vi "BasicMovement.vi"() -> ()   [LabVIEW 2015, in "IoTprojectg61305.lvrbt"]
uses:
  IoTprojectg61305.lvrbt
  <vilib>/NXT/Block Support/NXT_InputPort.ctl
  <vilib>/NXT/Block Support/NXT_OutputPort.ctl
  <vilib>/NXT/Dual Mode Library/Sensors/Touch_Pressed.vi
  <vilib>/NXT/Dual Mode Library/Sensors/EV3_Infrared_Proxy.vi
  <vilib>/NXT/NXTIO Xnodes/NXTIONodeSubVIs/NXTStopMotors.vi
  <vilib>/NXT/NXTIO Xnodes/NXTIONodeSubVIs/NXTMoveMotors.vi
  <vilib>/NXT/Dual Mode Library/Sound/Tone.vi
  <vilib>/NXT/Subs/LVHSConnector.ctl
  <vilib>/NXT/NXTIO Xnodes/AddressXNode/NXTIOAddress.xnode
  <vilib>/NXT/NXTIO Xnodes/NXTIOXNode/NXTIO.xnode
  <vilib>/NXT/LegoClasses/BrickReference/BrickReference.lvclass
panel:
  out "LEFT":bool
  out "STOP":bool
  out "OBSTACLE":bool
  out "posTab":i32
  in  "stop":bool
  out "RIGHT":bool
  out "new value":string
  out "old value":string
  out "UP":bool
  out "DOWN":bool
  # "Robot Modile Connecté : Lego Mindestrom EV3"
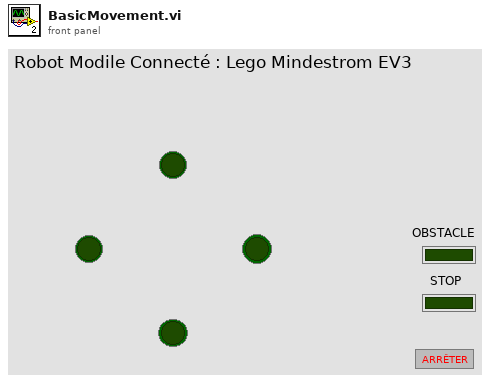
[diagram p1: front panel]
types:
  T1 = typedef "NXT_OutputPort.ctl" = u8
  T2 = typedef "NXT_InputPort.ctl" = u32
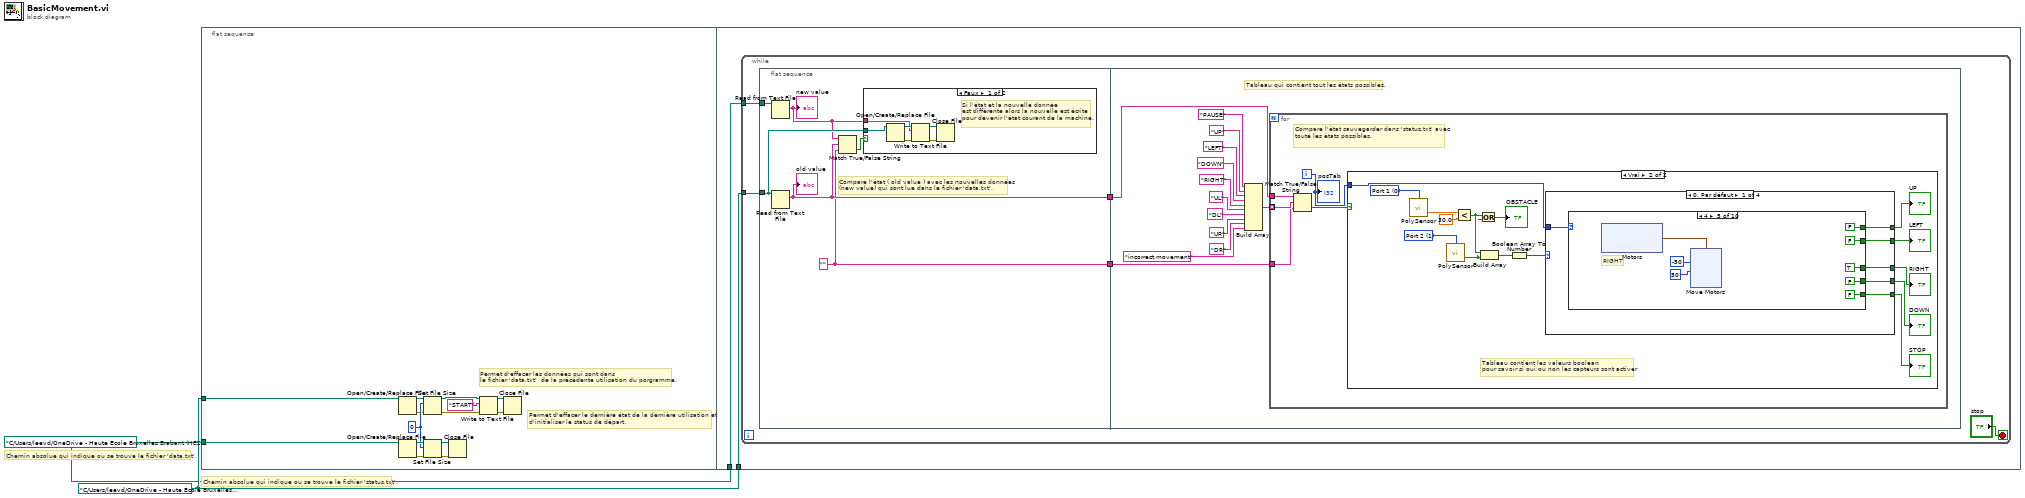
[diagram p0: block diagram]
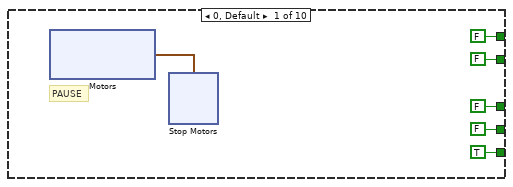
[diagram p4: hidden frame]
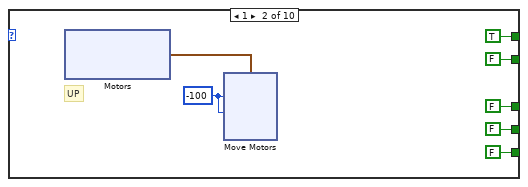
[diagram p5: hidden frame]
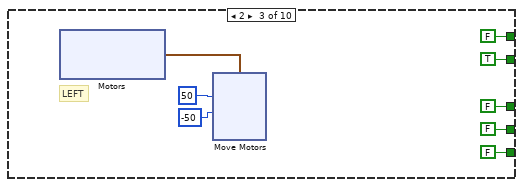
[diagram p6: hidden frame]
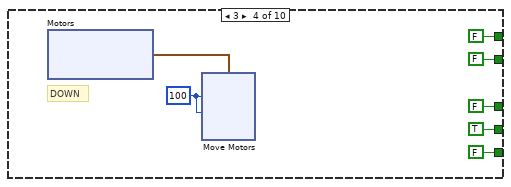
[diagram p7: hidden frame]
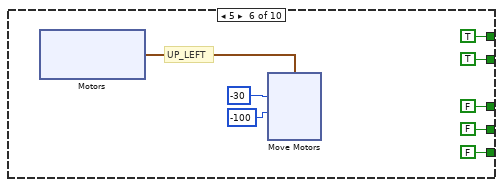
[diagram p8: hidden frame]
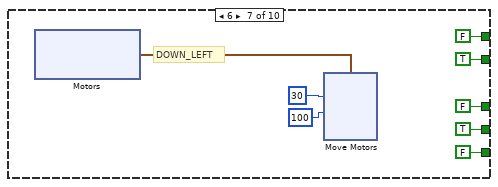
[diagram p9: hidden frame]
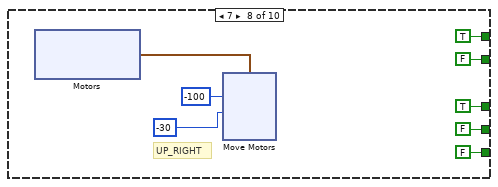
[diagram p10: hidden frame]
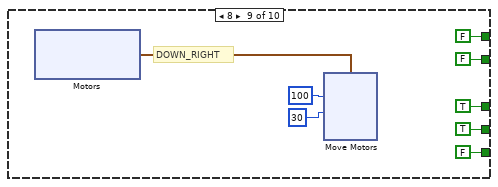
[diagram p11: hidden frame]
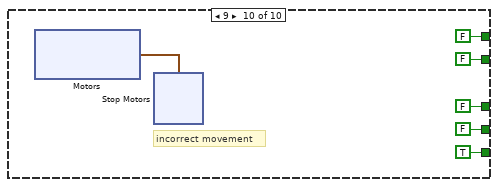
[diagram p12: hidden frame]
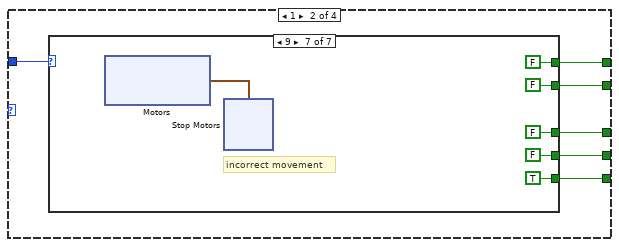
[diagram p13: hidden frame]
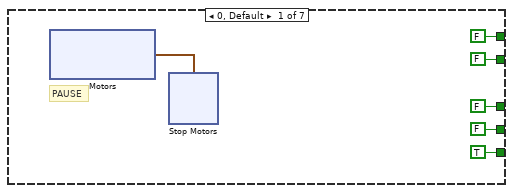
[diagram p14: hidden frame]
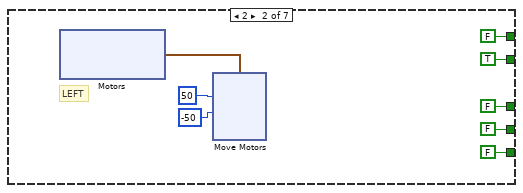
[diagram p15: hidden frame]
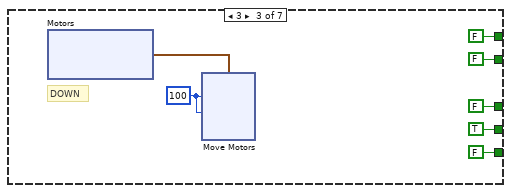
[diagram p16: hidden frame]
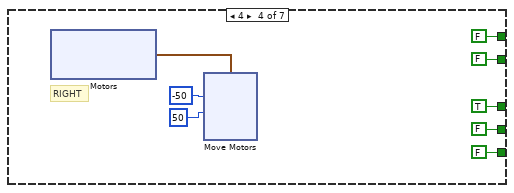
[diagram p17: hidden frame]
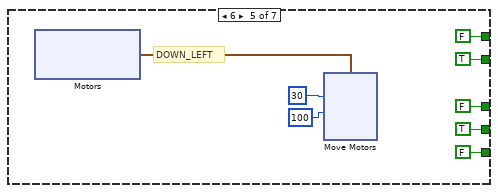
[diagram p18: hidden frame]
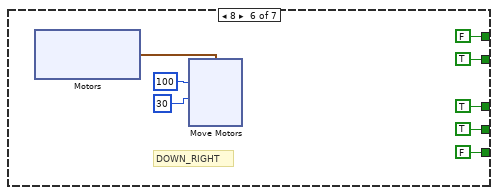
[diagram p19: hidden frame]
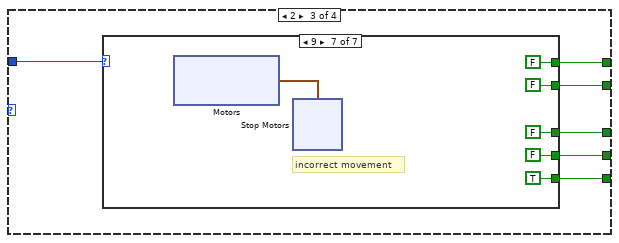
[diagram p20: hidden frame]
diagram:
  w2 = path "C:/Users/leevd/OneDrive - Haute Ecole Bruxelles Brabant (HE2B)/HE2B/Q4/IOTI4/Projet/HandTraking61305/data.txt" ("fichier (utiliser une boîte de dialogue)")
  w1 = path "C:/Users/leevd/OneDrive - Haute Ecole Bruxelles Brabant (HE2B)/HE2B/Q4/IOTI4/Projet/IoTprojectg61305/status.txt" ("fichier (utiliser une boîte de dialogue)")
  # "Chemin absolue qui indique ou se trouve le fichier 'status.txt'."
  # "Chemin absolue qui indique ou se trouve le fichier 'data.txt'."
  n1 = flat-sequence {
    tunnel: w2 -> [w9]
    tunnel: w1 -> [w8]
    tunnel: w1 -> [w17]
    tunnel: w2 -> [w18]
    frame #0 {
      w7 = i64 0 ("taille (en octets)")
      # "Permet d'effacer le dernière état de la dernière utilisation et \nd'initialiser le status de départ."
      # "Permet d'effacer les données qui sont dans \nle fichier 'data.txt'  de la précédente utilisation du porgramme."
      n2 = Open/Create/Replace File(file path (use dialog)=w9) -> (refnum out=w6:refnum<file>, error out=w3:errorcluster)  [unwired: 5 in, 1 out]
      n3 = Open/Create/Replace File(file path (use dialog)=w8) -> (refnum out=w15:refnum<file>, error out=w11:errorcluster)  [unwired: 5 in, 1 out]
      n4 = Set File Size(4:w3, 6:w7, 7:w6) -> (0:w4:errorcluster, 3:w5:refnum<file>)
      n5 = Set File Size(4:w11, 6:w7, 7:w15) -> (0:w12:errorcluster, 3:w13:refnum<file>)
      n6 = Close File(refnum=w13, error in=w12) -> ()  [unwired: 2 out]
      n7 = Write to Text File(file (use dialog)=w5, text="START", error in=w4) -> (refnum out=w14:refnum<file>, error out=w10:errorcluster)  [unwired: 1 in, 1 out]
      n8 = Close File(refnum=w14, error in=w10) -> ()  [unwired: 2 out]
    }
    frame #1 {
      n9 = while {
        tunnel: w18 -> [w22]
        tunnel: w17 -> [w21]
        stop <- "stop" stop-if-true
        n10 = flat-sequence {
          tunnel: w22 -> [w27]
          tunnel: w21 -> [w28]
          tunnel: [w25] -> w20
          tunnel: [w24] -> w19
          tunnel: w20 -> [w48]
          tunnel: w19 -> [w37]
          frame #0 {
            w24 = ""
            # "Compare l'état ( old value ) avec les nouvelles données\n(new value) qui sont lue dans le fichier 'data.txt'."
            n11 = Read from Text File(file (use dialog)=w28) -> (text=w26:string)  [unwired: 3 in, 3 out]
            "new value" <- w26
            n12 = Read from Text File(file (use dialog)=w27) -> (text=w25:string)  [unwired: 3 in, 3 out]
            "old value" <- w25
            n13 = Match True/False String(2:w24, 3:w25, 4:w26) -> (0:w29:bool)  [unwired: 1 out]
            n14 = case shown="Faux" w29 {
              tunnel: w26 -> [w31 _]
              tunnel: w27 -> [w30 _]
              frame False {
                # "Si l'état et la nouvelle donnée\nest différente alors la nouvelle est écrite \npour devenir l'état courant de la machine."
                n15 = Open/Create/Replace File(file path (use dialog)=w30) -> (refnum out=w35:refnum<file>, error out=w33:errorcluster)  [unwired: 5 in, 1 out]
                n16 = Write to Text File(file (use dialog)=w35, text=w31, error in=w33) -> (refnum out=w34:refnum<file>, error out=w32:errorcluster)  [unwired: 1 in, 1 out]
                n17 = Close File(refnum=w34, error in=w32) -> ()  [unwired: 2 out]
              }
              frame True {
              }
            }
          }
          frame #1 {
            # "Tableau qui contient tout les états possibles."
            n18 = Build Array("PAUSE", "UP", "LEFT", "DOWN", "RIGHT", "UL", "DL", "UR", "DR", "incorrect movement") -> (w47:string[])
            n19 = for {
              tunnel: w48 -> [w53]
              tunnel: w47 -> [w52] mode=indexing
              tunnel: w37 -> [w49]
              i -> [w50]
              # "Compare l'état sauvegarder dans 'status.txt' avec\ntoute les états possibles."
              n20 = Match True/False String(2:w49, 3:w52, 4:w53) -> (0:w51:bool)  [unwired: 1 out]
              n21 = case shown="Vrai" w51 {
                tunnel: w50 -> [_ w64]
                frame False {
                }
                frame True {
                  w67 = T2 0 items=["Port 1", "Port 2", "Port 3", "Port 4"] ("Port (Port 1)")
                  w68 = T2 1 items=["Port 1", "Port 2", "Port 3", "Port 4"] ("Port (Port 1)")
                  # "Tableau contient les valeurs boolean \npour savoir si oui ou non les capteurs sont activer"
                  n22 = call-poly <vilib>:"PolySensor.vi"("Port (Port 1)"=w67) -> ("Scaled Value"=w59:sgl)  [unwired: 2 in, 1 out]
                  n23 = call-poly <vilib>:"PolySensor.vi"("Port (Port 1)"=w68) -> ("Yes / No"=w56:bool)  [unwired: 2 in, 1 out]
                  n24 = Less?(x=w59, y=sgl 30.0) -> (x < y?=w57:bool)
                  n25 = Or(x=w57, y=w56) -> (x .or. y?=→"OBSTACLE":bool)
                  n26 = Build Array(w57, w56) -> (w66:bool[])
                  n27 = Boolean Array To Number(Boolean array=w66) -> (number=w65:u32)
                  n28 = case shown="0, Par défaut" w65 {
                    tunnel: w64 -> [w74 w233 w352 _]
                    tunnel: [w73 w237 w347 FALSE] -> w54
                    tunnel: [w72 w236 w348 FALSE] -> w63
                    tunnel: [w71 w235 w349 FALSE] -> w62
                    tunnel: [w70 w234 w350 FALSE] -> w61
                    tunnel: [w69 w238 w351 FALSE] -> w60
                    frame 0, Default {
                      n29 = case shown="4" w74 {
                        tunnel: [TRUE FALSE FALSE FALSE FALSE FALSE FALSE FALSE FALSE TRUE] -> w73
                        tunnel: [FALSE FALSE FALSE TRUE FALSE FALSE TRUE FALSE TRUE FALSE] -> w72
                        tunnel: [FALSE FALSE FALSE FALSE TRUE FALSE FALSE TRUE TRUE FALSE] -> w71
                        tunnel: [FALSE FALSE TRUE FALSE FALSE TRUE TRUE FALSE FALSE FALSE] -> w70
                        tunnel: [FALSE TRUE FALSE FALSE FALSE TRUE FALSE TRUE FALSE FALSE] -> w69
                        frame 0, Default {
                          # "PAUSE"
                          n30 = xnode "Motors"() -> ("Motor"=w80:cluster{"Port":T1, "Port":T1})
                          n31 = xnode "Stop Motors"("Motors"=w80) -> ()  [unwired: 1 in, 1 out]
                        }
                        frame 1 {
                          w93 = i8 -100 ("Power/Speed 2")
                          # "UP"
                          n32 = xnode "Motors"() -> ("Motor"=w92:cluster{"Port":T1, "Port":T1})
                          n33 = xnode "Move Motors"("Power/Speed 2"=w93, "Power/Speed 1"=w93, "Motors"=w92) -> ()  [unwired: 1 in, 1 out]
                        }
                        frame 2 {
                          # "LEFT"
                          n34 = xnode "Motors"() -> ("Motor"=w108:cluster{"Port":T1, "Port":T1})
                          n35 = xnode "Move Motors"("Power/Speed 2"=i8 -50, "Power/Speed 1"=i8 50 ("Power/Speed 2"), "Motors"=w108) -> ()  [unwired: 1 in, 1 out]
                        }
                        frame 3 {
                          w126 = i8 100 ("Power/Speed 2")
                          # "DOWN"
                          n36 = xnode "Motors"() -> ("Motor"=w125:cluster{"Port":T1, "Port":T1})
                          n37 = xnode "Move Motors"("Power/Speed 2"=w126, "Power/Speed 1"=w126, "Motors"=w125) -> ()  [unwired: 1 in, 1 out]
                        }
                        frame 4 {
                          # "RIGHT"
                          n38 = xnode "Motors"() -> ("Motor"=w141:cluster{"Port":T1, "Port":T1})
                          n39 = xnode "Move Motors"("Power/Speed 2"=i8 50, "Power/Speed 1"=i8 -50 ("Power/Speed 2"), "Motors"=w141) -> ()  [unwired: 1 in, 1 out]
                        }
                        frame 5 {
                          # "UP_LEFT"
                          n40 = xnode "Motors"() -> ("Motor"=w158:cluster{"Port":T1, "Port":T1})
                          n41 = xnode "Move Motors"("Power/Speed 2"=i8 -100, "Power/Speed 1"=i8 -30 ("Power/Speed 2"), "Motors"=w158) -> ()  [unwired: 1 in, 1 out]
                        }
                        frame 6 {
                          # "DOWN_LEFT"
                          n42 = xnode "Motors"() -> ("Motor"=w175:cluster{"Port":T1, "Port":T1})
                          n43 = xnode "Move Motors"("Power/Speed 2"=i8 100, "Power/Speed 1"=i8 30 ("Power/Speed 2"), "Motors"=w175) -> ()  [unwired: 1 in, 1 out]
                        }
                        frame 7 {
                          # "UP_RIGHT"
                          n44 = xnode "Motors"() -> ("Motor"=w192:cluster{"Port":T1, "Port":T1})
                          n45 = xnode "Move Motors"("Power/Speed 2"=i8 -30, "Power/Speed 1"=i8 -100 ("Power/Speed 2"), "Motors"=w192) -> ()  [unwired: 1 in, 1 out]
                        }
                        frame 8 {
                          # "DOWN_RIGHT"
                          n46 = xnode "Motors"() -> ("Motor"=w209:cluster{"Port":T1, "Port":T1})
                          n47 = xnode "Move Motors"("Power/Speed 2"=i8 30, "Power/Speed 1"=i8 100 ("Power/Speed 2"), "Motors"=w209) -> ()  [unwired: 1 in, 1 out]
                        }
                        frame 9 {
                          # "incorrect movement"
                          n48 = xnode "Motors"() -> ("Motor"=w226:cluster{"Port":T1, "Port":T1})
                          n49 = xnode "Stop Motors"("Motors"=w226) -> ()  [unwired: 1 in, 1 out]
                        }
                      }
                    }
                    frame 1 {
                      n50 = case shown="9" w233 {
                        tunnel: [FALSE FALSE FALSE FALSE FALSE FALSE FALSE] -> w238
                        tunnel: [TRUE FALSE FALSE FALSE FALSE FALSE TRUE] -> w237
                        tunnel: [FALSE FALSE TRUE FALSE TRUE TRUE FALSE] -> w236
                        tunnel: [FALSE FALSE FALSE TRUE FALSE TRUE FALSE] -> w235
                        tunnel: [FALSE TRUE FALSE FALSE TRUE TRUE FALSE] -> w234
                        frame 0, Default {
                          # "PAUSE"
                          n51 = xnode "Motors"() -> ("Motor"=w244:cluster{"Port":T1, "Port":T1})
                          n52 = xnode "Stop Motors"("Motors"=w244) -> ()  [unwired: 1 in, 1 out]
                        }
                        frame 2 {
                          # "LEFT"
                          n53 = xnode "Motors"() -> ("Motor"=w256:cluster{"Port":T1, "Port":T1})
                          n54 = xnode "Move Motors"("Power/Speed 2"=i8 -50, "Power/Speed 1"=i8 50 ("Power/Speed 2"), "Motors"=w256) -> ()  [unwired: 1 in, 1 out]
                        }
                        frame 3 {
                          w274 = i8 100 ("Power/Speed 2")
                          # "DOWN"
                          n55 = xnode "Motors"() -> ("Motor"=w273:cluster{"Port":T1, "Port":T1})
                          n56 = xnode "Move Motors"("Power/Speed 2"=w274, "Power/Speed 1"=w274, "Motors"=w273) -> ()  [unwired: 1 in, 1 out]
                        }
                        frame 4 {
                          # "RIGHT"
                          n57 = xnode "Motors"() -> ("Motor"=w289:cluster{"Port":T1, "Port":T1})
                          n58 = xnode "Move Motors"("Power/Speed 2"=i8 50, "Power/Speed 1"=i8 -50 ("Power/Speed 2"), "Motors"=w289) -> ()  [unwired: 1 in, 1 out]
                        }
                        frame 6 {
                          # "DOWN_LEFT"
                          n59 = xnode "Motors"() -> ("Motor"=w306:cluster{"Port":T1, "Port":T1})
                          n60 = xnode "Move Motors"("Power/Speed 2"=i8 100, "Power/Speed 1"=i8 30 ("Power/Speed 2"), "Motors"=w306) -> ()  [unwired: 1 in, 1 out]
                        }
                        frame 8 {
                          # "DOWN_RIGHT"
                          n61 = xnode "Motors"() -> ("Motor"=w323:cluster{"Port":T1, "Port":T1})
                          n62 = xnode "Move Motors"("Power/Speed 2"=i8 30, "Power/Speed 1"=i8 100 ("Power/Speed 2"), "Motors"=w323) -> ()  [unwired: 1 in, 1 out]
                        }
                        frame 9 {
                          # "incorrect movement"
                          n63 = xnode "Motors"() -> ("Motor"=w340:cluster{"Port":T1, "Port":T1})
                          n64 = xnode "Stop Motors"("Motors"=w340) -> ()  [unwired: 1 in, 1 out]
                        }
                      }
                    }
                    frame 2 {
                      n65 = case shown="9" w352 {
                        tunnel: [FALSE TRUE FALSE FALSE TRUE TRUE FALSE] -> w351
                        tunnel: [FALSE FALSE TRUE FALSE TRUE FALSE FALSE] -> w350
                        tunnel: [FALSE FALSE FALSE TRUE TRUE TRUE FALSE] -> w349
                        tunnel: [FALSE FALSE FALSE FALSE FALSE FALSE FALSE] -> w348
                        tunnel: [TRUE FALSE FALSE FALSE FALSE FALSE TRUE] -> w347
                        frame 0, Default {
                          # "PAUSE"
                          n66 = xnode "Motors"() -> ("Motor"=w358:cluster{"Port":T1, "Port":T1})
                          n67 = xnode "Stop Motors"("Motors"=w358) -> ()  [unwired: 1 in, 1 out]
                        }
                        frame 1 {
                          w371 = i8 -100 ("Power/Speed 2")
                          # "UP"
                          n68 = xnode "Motors"() -> ("Motor"=w370:cluster{"Port":T1, "Port":T1})
                          n69 = xnode "Move Motors"("Power/Speed 2"=w371, "Power/Speed 1"=w371, "Motors"=w370) -> ()  [unwired: 1 in, 1 out]
                        }
                        frame 2 {
                          # "LEFT"
                          n70 = xnode "Motors"() -> ("Motor"=w386:cluster{"Port":T1, "Port":T1})
                          n71 = xnode "Move Motors"("Power/Speed 2"=i8 -50, "Power/Speed 1"=i8 50 ("Power/Speed 2"), "Motors"=w386) -> ()  [unwired: 1 in, 1 out]
                        }
                        frame 4 {
                          # "RIGHT"
                          n72 = xnode "Motors"() -> ("Motor"=w403:cluster{"Port":T1, "Port":T1})
                          n73 = xnode "Move Motors"("Power/Speed 2"=i8 50, "Power/Speed 1"=i8 -50 ("Power/Speed 2"), "Motors"=w403) -> ()  [unwired: 1 in, 1 out]
                        }
                        frame 5 {
                          # "UP_LEFT"
                          n74 = xnode "Motors"() -> ("Motor"=w420:cluster{"Port":T1, "Port":T1})
                          n75 = xnode "Move Motors"("Power/Speed 2"=i8 -100, "Power/Speed 1"=i8 -30 ("Power/Speed 2"), "Motors"=w420) -> ()  [unwired: 1 in, 1 out]
                        }
                        frame 7 {
                          # "UP_RIGHT"
                          n76 = xnode "Motors"() -> ("Motor"=w437:cluster{"Port":T1, "Port":T1})
                          n77 = xnode "Move Motors"("Power/Speed 2"=i8 -30, "Power/Speed 1"=i8 -100 ("Power/Speed 2"), "Motors"=w437) -> ()  [unwired: 1 in, 1 out]
                        }
                        frame 9 {
                          # "incorrect movement"
                          n78 = xnode "Motors"() -> ("Motor"=w454:cluster{"Port":T1, "Port":T1})
                          n79 = xnode "Stop Motors"("Motors"=w454) -> ()  [unwired: 1 in, 1 out]
                        }
                      }
                    }
                    frame 3 {
                      n80 = call-poly <vilib>:"PolySound.vi"() -> ()  [unwired: 4 in, 1 out]
                    }
                  }
                  "UP" <- w60
                  "DOWN" <- w63
                  "LEFT" <- w61
                  "RIGHT" <- w62
                  "STOP" <- w54
                }
              }
              "posTab" <- w50
            }
          }
        }
      }
    }
  }
